vi "FirstOrderSys.vi"() -> ()   [LabVIEW 2015]
panel:
  in  "Stop Button":bool
  out "Settling Time (Ts)":dbl[](array[numeric])
  out "Rise Time (Tr)":dbl[](array[numeric])
  out "Time Delay (Td)":dbl
  in  "Time constant":dbl(slide) scale=0.0..10.0
  out "Waveform Chart":cluster{dbl, dbl}(graph)
  # "Time Response"
  # "First Order System"
  # "s"
  # "s"
  # "s"
  # "s"
  # "s"
  # "s"
  # "Tr (5% - 95%)"
  # "Tr (10% - 90%)"
  # "Ts (+- 0.5%)"
  # "Ts (+- 2%)"
  # "Ts (+- 3%)"
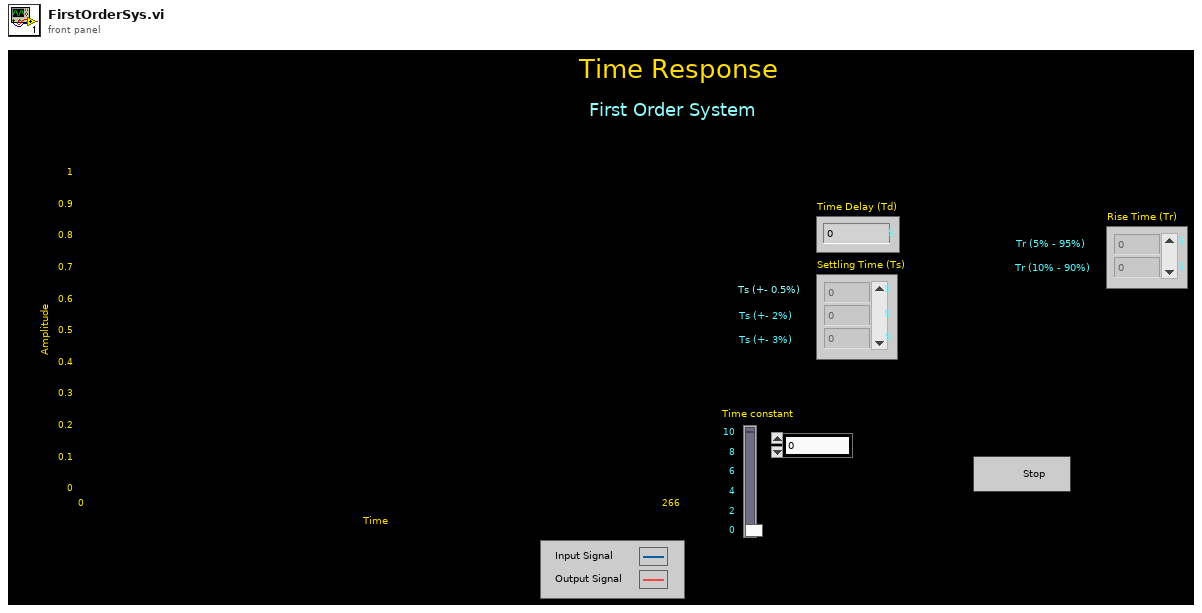
[diagram p1: front panel]
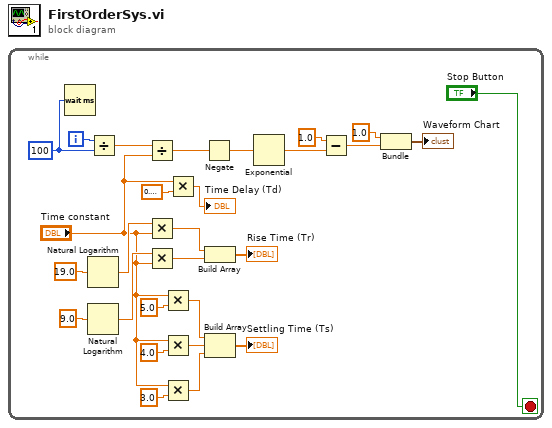
[diagram p0: block diagram]
diagram:
  n1 = while {
    i -> [w28]
    stop <- "Stop Button" stop-if-true
    w27 = 100 ("y")
    n2 = Wait (ms)(milliseconds to wait=w27) -> ()  [unwired: 1 out]
    n3 = Natural Logarithm(1:19.0 ("x")) -> (0:w15:dbl)
    n4 = Natural Logarithm(1:9.0 ("x")) -> (0:w11:dbl)
    n5 = Divide(x=w28, y=w27) -> (x/y=w26:dbl)
    n6 = Divide(x=w26, y="Time constant") -> (x/y=w25:dbl)
    n7 = Multiply(x=w15, y="Time constant") -> (x*y=w14:dbl)
    n8 = Multiply(x=w11, y="Time constant") -> (x*y=w10:dbl)
    n9 = Multiply(x="Time constant", y=5.0) -> (x*y=w7:dbl)
    n10 = Multiply(x="Time constant", y=4.0) -> (x*y=w5:dbl)
    n11 = Multiply(x="Time constant", y=3.0) -> (x*y=w4:dbl)
    n12 = Multiply(x="Time constant", y=0.6931471805599453) -> (x*y=→"Time Delay (Td)":dbl)
    n13 = Negate(x=w25) -> (-x=w24:dbl)
    n14 = Build Array(w14, w10) -> (→"Rise Time (Tr)":dbl[])
    n15 = Build Array(w7, w5, w4) -> (→"Settling Time (Ts)":dbl[])
    n16 = Exponential(1:w24) -> (0:w23:dbl)
    n17 = Subtract(x=1.0, y=w23) -> (x-y=w21:dbl)
    n18 = Bundle(1.0, w21) -> (→"Waveform Chart":cluster{dbl, dbl})  [unwired: 1 in]
  }
